vi "Read_Measurements.vi"(8 "error in (no error)":errorcluster, 11 "BMP208 in":refnum<class "BMP208.lvclass">) -> (0 "error out":errorcluster, 2 "Measurements":T1, 3 "BMP208 out":refnum<class "BMP208.lvclass">)   [LabVIEW 2020, in "BMP208.lvclass"]
uses:
  BMP208.lvclass
  Controls/td_cluster_measurements.ctl
  BMP208.lvclass/BMP208.ctl
  Properties/Read TempCoeff.vi
  Properties/Read PressCoeff.vi
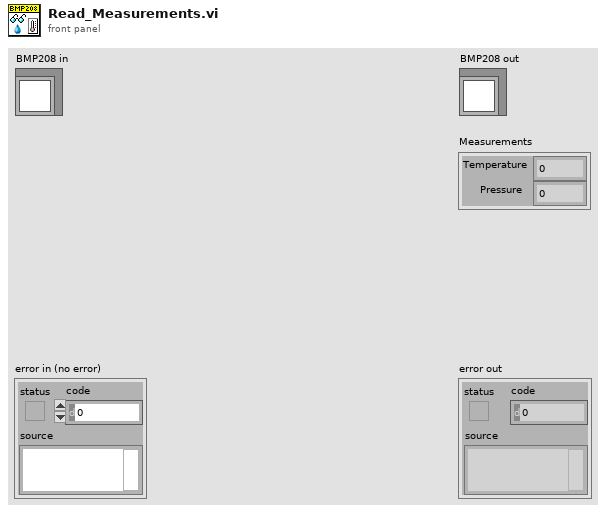
[diagram p1: front panel]
types:
  T1 = typedef "BMP208.lvclass/td_cluster_measurements.ctl" = cluster{"Temperature":dbl, "Pressure":dbl}
  T2 = typedef "BMP208.lvclass/td_cluster_Temp_Coeff.ctl" = cluster{"T1":u16, "T2":i16, "T3":i16}
  T3 = typedef "BMP208.lvclass/td_cluster_Press_Coeff.ctl" = cluster{"P1":u16, "P2":i16, "P3":i16, "P4":i16, "P5":i16, "P6":i16, "P7":i16, "P8":i16, "P9":i16}
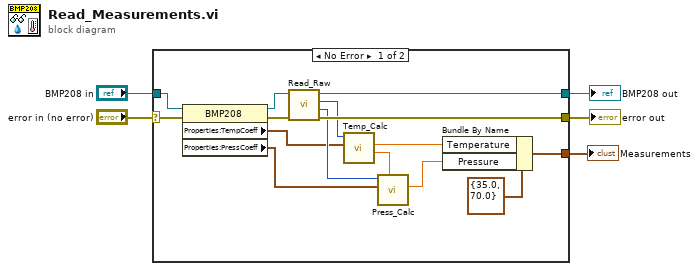
[diagram p0: block diagram]
diagram:
  n1 = case shown="No Error" "error in (no error)" {
    selector: "error in (no error)" -> [w17 w22]
    tunnel: [w14 w22] -> w4
    tunnel: [w12 w21] -> w2
    tunnel: "BMP208 in" -> [w15 w21]
    tunnel: [w19 _] -> w1
    frame No Error {
      n2 = property class="BMP208"(reference=w15, error in=w17) -> (reference out=w13:refnum<class "BMP208.lvclass">, error out=w16:errorcluster, "Properties:TempCoeff"=w9:T2, "Properties:PressCoeff"=w8:T3)
      n3 = call "Read_Raw.vi"("error in (no error)"=w16, "BMP208 in"=w13) -> ("error out"=w14:errorcluster, "PressureU32"=w10:u32, "TempU32"=w11:u32, "BMP208 out"=w12:refnum<class "BMP208.lvclass">)  [unwired: 6 in]
      n4 = call "Temp_Calc.vi"("TempCoeff"=w9, "raw_temp"=w11) -> ("tfine"=w6:dbl, "Temperature"=w18:dbl)  [unwired: 8 in]
      n5 = call "Press_Calc.vi"("tfine"=w6, "PressCoeff"=w8, "PressureReadingU32"=w10) -> ("Pressure(Pa)"=w7:dbl)  [unwired: 8 in]
      n6 = Bundle By Name(cluster=T1 {"Temperature"=35.0, "Pressure"=70.0} ("Measurements"), "Temperature"=w18, "Pressure"=w7) -> (w19:T1)
    }
    frame Error {
    }
  }
  "error out" <- w4
  "BMP208 out" <- w2
  "Measurements" <- w1
